vi "Translation3d_Minus.vi"(9 "other Translation3d":T1 {"Z" format="%14.3f"; "Y" format="%14.3f"; "X" format="%14.3f"}, 11 "In Translation3d":T1 {"Z" format="%14.3f"; "Y" format="%14.3f"; "X" format="%14.3f"}) -> (3 "Out Translation3d":T1 {"Z" format="%14.3f"; "Y" format="%14.3f"; "X" format="%14.3f"})   [LabVIEW 2019, in "Trajectory_Library.lvlib"]
doc: "Returns the difference between two translations.\n \nFor example, Translation3d(5.0, 4.0, 3.0) - Translation3d(1.0, 2.0, 3.0) = Translation3d(4.0, 2.0, 0.0).\n\nParameters:\n - IN Translation3d - This translation3d data structure\n - other Translation3d - The translation3d data structure to subtract\n\nReturns\n - Out Translation3d - The difference between the two translations."
uses:
  Trajectory_Library.lvlib
  TypeDef/TRANSLATION3D.ctl
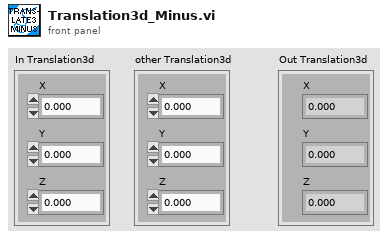
[diagram p1: front panel]
types:
  T1 = typedef "Trajectory_Library.lvlib/TRANSLATION3D.ctl" = cluster{"X":dbl, "Y":dbl, "Z":dbl}
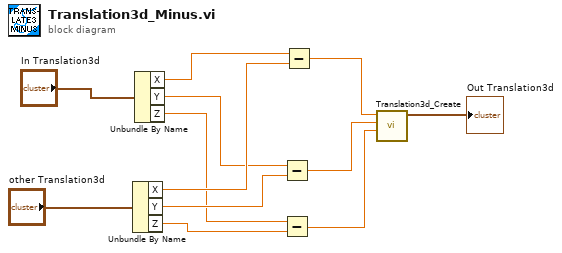
[diagram p0: block diagram]
diagram:
  n1 = Unbundle By Name("other Translation3d") -> ("X"=w9:dbl, "Y"=w4:dbl, "Z"=w2:dbl)
  n2 = Unbundle By Name("In Translation3d") -> ("X"=w10:dbl, "Y"=w8:dbl, "Z"=w3:dbl)
  n3 = Subtract(x=w8, y=w4) -> (x-y=w5:dbl)
  n4 = Subtract(x=w3, y=w2) -> (x-y=w1:dbl)
  n5 = Subtract(x=w10, y=w9) -> (x-y=w6:dbl)
  n6 = call "Translation3d_Create.vi"("Z"=w1, "Y"=w5, "X"=w6) -> ("TRANSLATION3D"=→"Out Translation3d":T1)  [unwired: 8 in]
